vi "subViAligo_8channel_display_legacy.vi"(4 "error in":errorcluster, 6 "Input":T2={"Digital Start Trigger Source 4"="/Dev1/PFI0", "Digital Start Trigger Edge 4"=10280, "minimum value"=-10.0, "maximum value"=10.0, "rate"=1000.0, "device name"="PXI1Slot5", "formular in"=[], "Total time"=0.0} {"rate" format="%0.2f"; "maximum value" format="%0.2f"; "minimum value" format="%0.2f"; "Digital Start Trigger Edge 4" items=["Rising"=10280, "Falling"=10171]}) -> (0 "error out":errorcluster, 2 "Output":T1={"Actual Rate"=0.0, "Actual SampPerChan"=0.0, "Mixed Signal Graph"=[], "模拟隔离器连接状态"="未连接模拟隔离器"}, 3 "task out":refnum<k21>)   [LabVIEW 2021]
uses:
  <resource>/objmgr/daqmx.rc
  <vilib>/DAQmx/create/channels.llb/DAQmx Create Channel (AO-Voltage-Basic).vi
  <vilib>/DAQmx/configure/trigger.llb/DAQmx Start Trigger (Digital Edge).vi
  <vilib>/DAQmx/configure/timing.llb/DAQmx Timing (Sample Clock).vi
  <vilib>/DAQmx/write.llb/DAQmx Write (Analog 1D Wfm NChan NSamp).vi
panel:
  # "1、模拟隔离器连接状态会根据\n你所选择的device name 来显\n示对应板卡的连接状态。\n2、Actual Rate显示实际的时钟\n频率。\n3、Actual SampPer Chan显示\n每次采样的总样本点数。\n4、由于模拟隔离芯片存在offset\n所以刚启动NI板卡时会存在100mv\n的offset，一旦触发运行之后会自动\n调节，offset也将不存在了。因此触发\n之后的实际电压以面板所显示的值为准。"
  # "1、formular in 中sample为各个分段函数的持续时间。\n2、Total time 为总时间，必须大于sample加起来的值。\n3、minimum value和maximum value默认±10V不改。\n4、rate为采样率，即时钟频率\n5、device name为选择的板卡名字，可选为PXI1Slot5-7\n6、Source 为接受触发的端口，Edge为选择上升沿触发\n还是其他类型触发。"
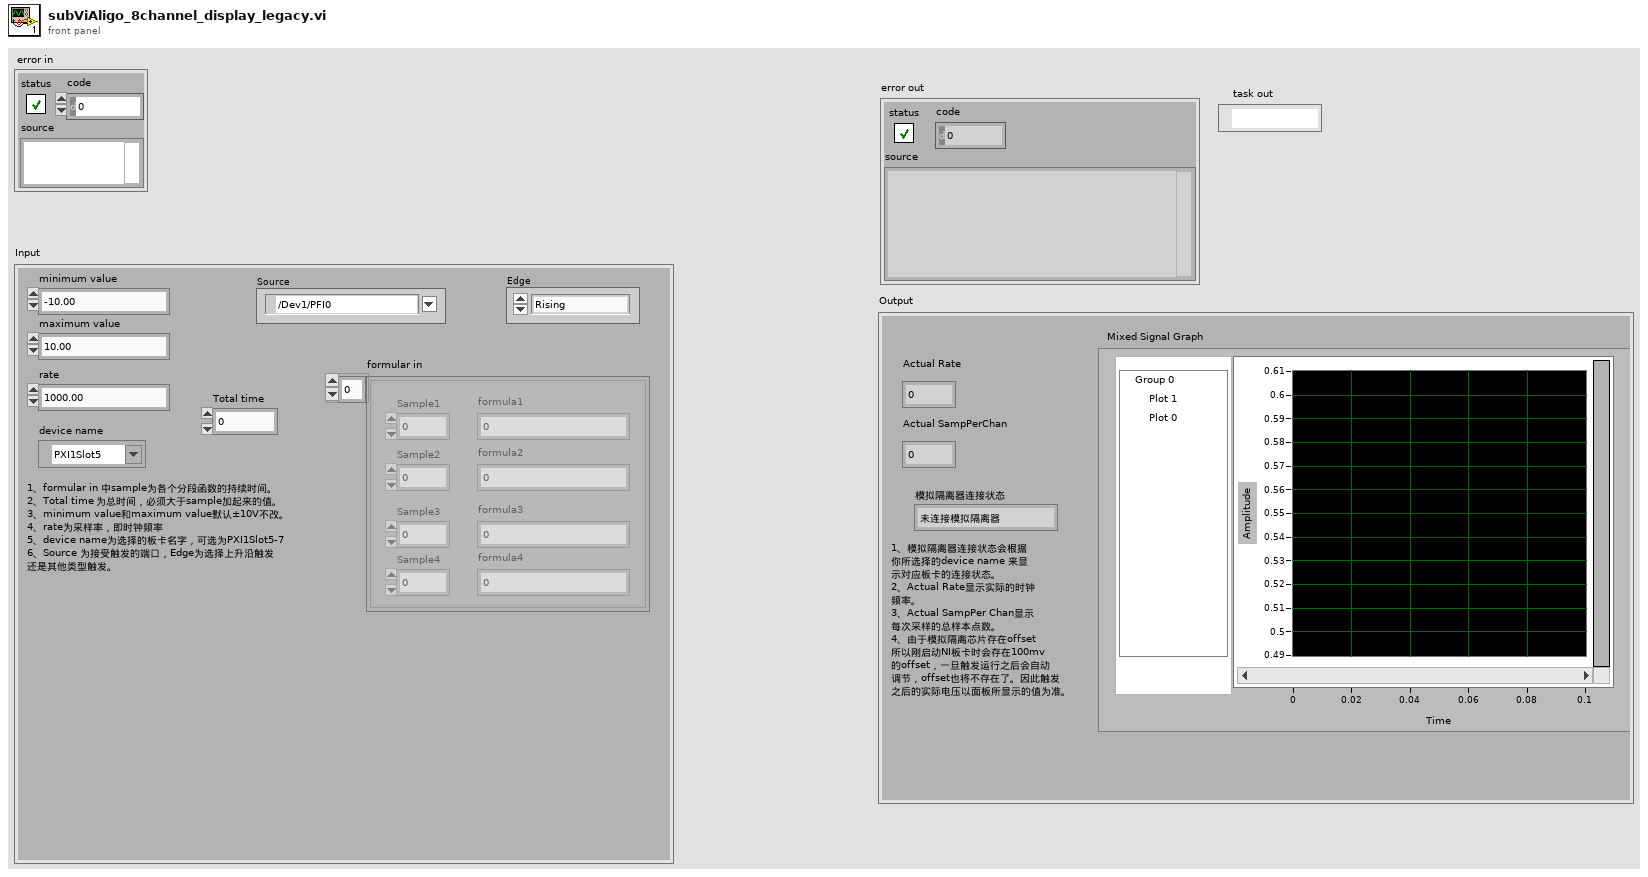
[diagram p1: front panel]
types:
  T1 = cluster{"Actual Rate":dbl, "Actual SampPerChan":dbl, "Mixed Signal Graph":waveform(dbl)[], "模拟隔离器连接状态":string}
  T2 = cluster{"Digital Start Trigger Source 4":tag, "Digital Start Trigger Edge 4":i32, "minimum value":dbl, "maximum value":dbl, "rate":dbl, "device name":tag, "formular in":cluster{"Sample1":dbl, "formula1":string, "Sample2":dbl, "formula2":string, "Sample3":dbl, "formula3":string, "Sample4":dbl, "formula4":string}[], "Total time":dbl}
  T3 = cluster{"Sample1":dbl, "formula1":string, "Sample2":dbl, "formula2":string, "Sample3":dbl, "formula3":string, "Sample4":dbl, "formula4":string}[]
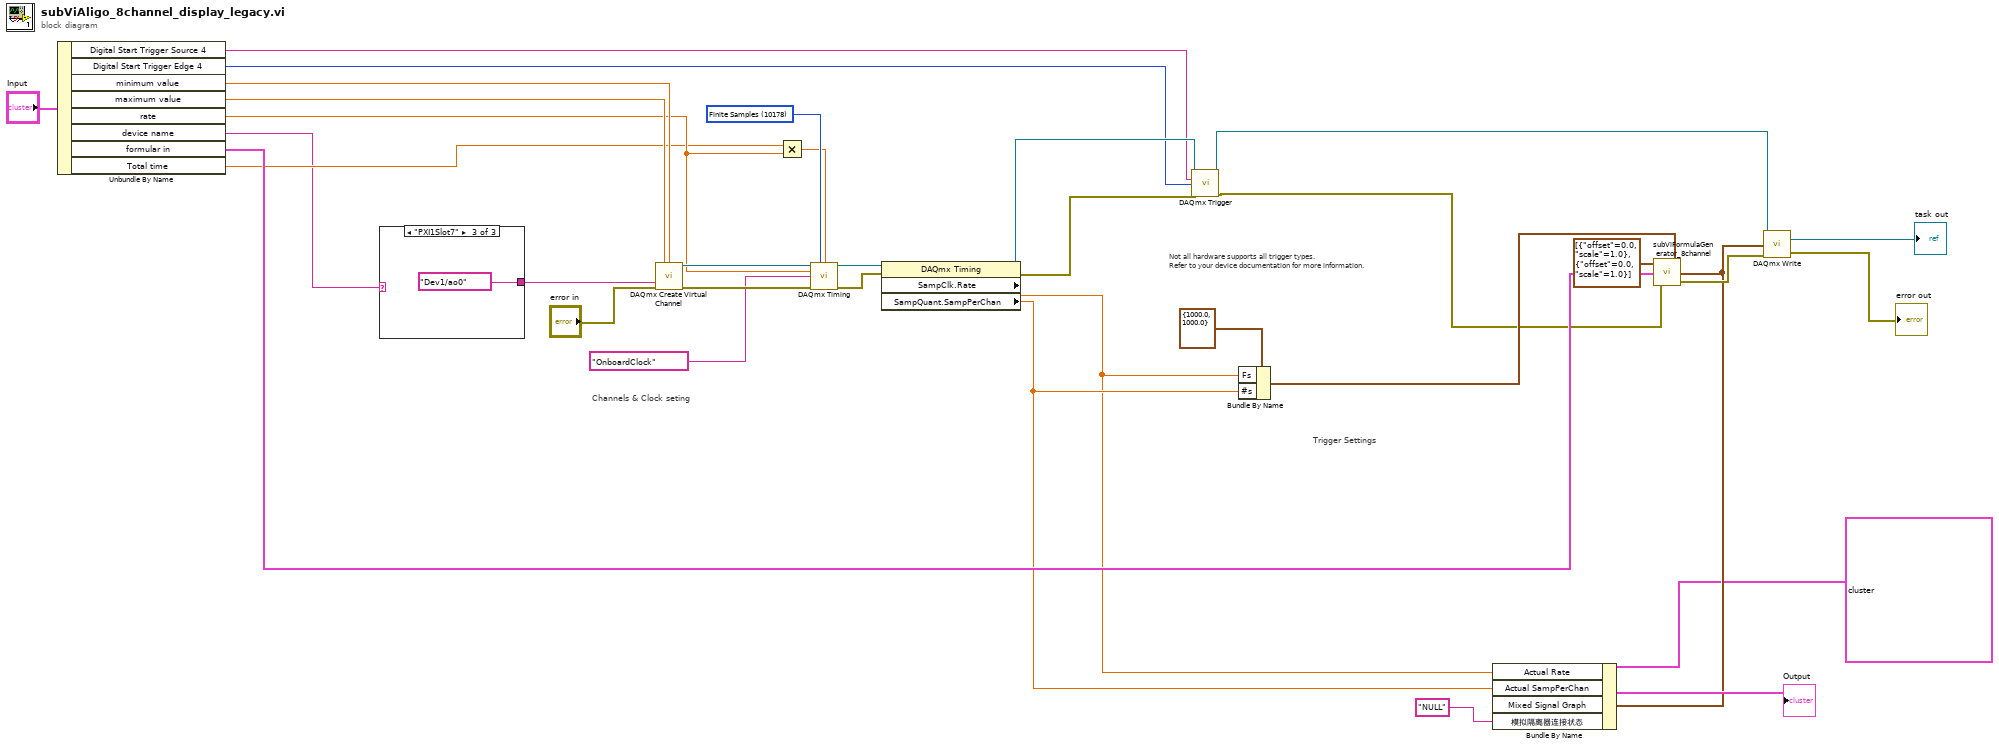
[diagram p0: block diagram]
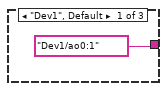
[diagram p2: hidden frame]
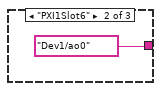
[diagram p3: hidden frame]
diagram:
  w34 = 10178 items=["Finite Samples"=10178, "Continuous Samples"=10123, "Hardware Timed Single Point"=12522] ("sample mode")
  # "Channels & Clock seting"
  # "Trigger Settings"
  # "Not all hardware supports all trigger types.\nRefer to your device documentation for more information."
  n1 = Unbundle By Name("Input") -> ("Digital Start Trigger Source 4"=w12:tag, "Digital Start Trigger Edge 4"=w11:i32, "minimum value"=w23:dbl, "maximum value"=w22:dbl, "rate"=w21:dbl, "device name"=w1:tag, "formular in"=w19:T3, "Total time"=w8:dbl)
  n2 = case shown="\"PXI1Slot7\"" w1 {
    tunnel: [tag "Dev1/ao0:1" ("physical channels") tag "Dev1/ao0" ("physical channels") tag "Dev1/ao0" ("physical channels")] -> w25
    frame "Dev1", Default {
    }
    frame "PXI1Slot6" {
    }
    frame "PXI1Slot7" {
    }
  }
  n3 = call-poly <vilib>:"DAQmx Create Virtual Channel.vi"("maximum value"=w22, "minimum value"=w23, "physical channels"=w25, "error in"="error in") -> ("task out"=w33:refnum<k21>, "error out"=w32:errorcluster)  [unwired: 10 in]
  n4 = Multiply(x=w8, y=w21) -> (x*y=w28:dbl)
  n5 = call-poly <vilib>:"DAQmx Timing.vi"("task/channels in"=w33, "sample mode"=w34, "samples per channel"=w28, "rate"=w21, "source"=tag "OnboardClock", "error in"=w32) -> ("task out"=w31:refnum<k21>, "error out"=w30:errorcluster)  [unwired: 8 in]
  n6 = property class="DAQmx Timing"(reference=w31, error in=w30) -> (reference out=w17:refnum<k21>, error out=w16:errorcluster, "SampClk.Rate"=w7:dbl, "SampQuant.SampPerChan"=w9:dbl)
  n7 = call-poly <vilib>:"DAQmx Trigger.vi"("task/channels in"=w17, "source"=w12, "edge"=w11, "error in"=w16) -> ("task out"=w18:refnum<k21>, "error out"=w4:errorcluster)  [unwired: 10 in]
  n8 = Bundle By Name(cluster=cluster{"Fs":dbl, "#s":dbl} {"Fs"=1000.0, "#s"=1000.0} ("sampling info"), "Fs"=w7, "#s"=w9) -> (w27:cluster{"Fs":dbl, "#s":dbl})
  n9 = call "subViFormulaGenerator_8channel.vi"("sampling info"=w27, "error in (no error)"=w4, "formular in"=w19, "regulatorArray"=cluster{"offset":dbl, "scale":dbl}[] [{"offset"=0.0, "scale"=1.0}, {"offset"=0.0, "scale"=1.0}]) -> ("error out"=w26:errorcluster, "formular out"=w15:waveform(dbl)[])
  n10 = Bundle By Name(cluster=T1 {"Actual Rate"=1000.0, "Actual SampPerChan"=2000.0, "Mixed Signal Graph"=[{"t0"=timestamp(0 s since 1904-01-01), "dt"=0.001, "Y"=array[2000 elements]}, {"t0"=timestamp(0 s since 1904-01-01), "dt"=0.001, "Y"=array[2000 elements]}, {"t0"=timestamp(0 s since 1904-01-01), "dt"=0.001, "Y"=array[2000 elements]}, {"t0"=timestamp(0 s since 1904-01-01), "dt"=0.001, "Y"=array[2000 elements]}, {"t0"=timestamp(0 s since 1904-01-01), "dt"=0.001, "Y"=array[2000 elements]}, {"t0"=timestamp(0 s since 1904-01-01), "dt"=0.001, "Y"=array[2000 elements]}, {"t0"=timestamp(0 s since 1904-01-01), "dt"=0.001, "Y"=array[2000 elements]}, {"t0"=timestamp(0 s since 1904-01-01), "dt"=0.001, "Y"=array[2000 elements]}], "模拟隔离器连接状态"="已连接1号模拟隔离器"} ("Cluster 2"), "Actual Rate"=w7, "Actual SampPerChan"=w9, "Mixed Signal Graph"=w15, "模拟隔离器连接状态"="NULL") -> (→"Output":T1)
  n11 = call-poly <vilib>:"DAQmx Write.vi"("task/channels in"=w18, "data"=w15, "error in"=w26) -> ("task out"=→"task out":refnum<k21>, "error out"=→"error out":errorcluster)  [unwired: 10 in, 1 out]
